vi "ave.vi"() -> ()   [LabVIEW 2015]
panel:
  out "Numeric 3":dbl
  in  "Numeric 2":dbl
  in  "Numeric":dbl
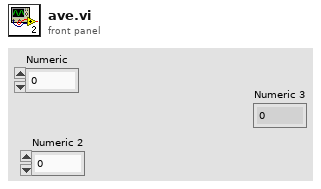
[diagram p1: front panel]
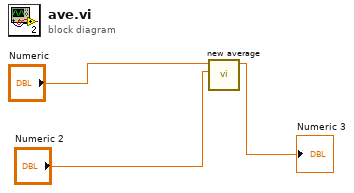
[diagram p0: block diagram]
diagram:
  n1 = call "new average.vi"("Numeric 3"="Numeric 2", "Numeric in"="Numeric") -> ("Numeric out"=→"Numeric 3":dbl)  [unwired: 9 in]
